vi "Set Matrix - file.vi"(5 "double array":dbl[][](array[numeric]), 6 "cmplx double array":cdb[][](array[numeric]), 7 "string array":string[](array[string]), 8 "error in (no error)":errorcluster, 10 "variable name":string, 11 "GOLPI ref. in":T1={"pipe handle"={"lv_proc.dll file path"=path "", "process instance handle"=[]}, "fast read timeout [ms]"=500, "fast read settle time [ms]"=10, "fast read to multiple [ms]"=1, "max elements per input line"=100}) -> (0 "error out":errorcluster, 3 "GOLPI ref. out":T1={"pipe handle"={"lv_proc.dll file path"=path "", "process instance handle"=[]}, "fast read timeout [ms]"=500, "fast read settle time [ms]"=10, "fast read to multiple [ms]"=1, "max elements per input line"=100})   [LabVIEW 2013, in "GOLPI library.lvlib"]
uses:
  GOLPI library.lvlib
  Type Definitions/GOLPI reference Type Def.ctl
  LV Process.lvlibp/Pipe Handle.ctl
  Type Definitions/Custom Error Codes Enum Type Def.vi
  LV Process.lvlibp
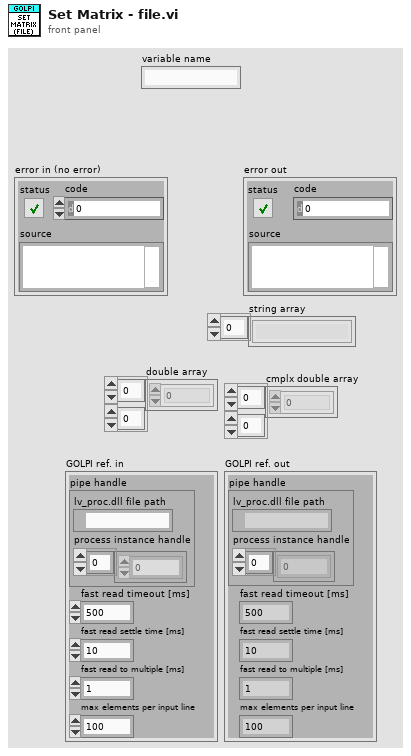
[diagram p1: front panel]
types:
  T1 = typedef "GOLPI library.lvlib/GOLPI reference Type Def.ctl" = cluster{"pipe handle":T2, "fast read timeout [ms]":u32, "fast read settle time [ms]":u32, "fast read to multiple [ms]":u32, "max elements per input line":u32}
  T2 = typedef "LV Process.lvlibp/Pipe Handle.ctl" = cluster{"lv_proc.dll file path":path, "process instance handle":u32[]}
  T3 = typedef "GOLPI library.lvlib/Custom Error Codes Enum Type Def.vi" = enum16{"no error", "00 working directory PAR1 missing", "01 octave binary PAR1 missing", "02 octave report error PAR1", "03 empty output last cmd PAR1", "04 missing temporary file PAR1", "05 pwd PAR 1 not exist", "10 var PAR1 not string", "11 var PAR1 not num, scal, ~compl", "12 var PAR1 not num, scal, compl", "13 var PAR1 not num, vect, ~compl", "14 var PAR1 not num, vect, compl", "15 var PAR1 not num, mat, ~compl", "16 var PAR1 not num, mat, ~compl", "99 not finished"}
  T4 = enum16{"open", "replace", "create", "open or create", "replace or create", "replace or create with confirmation"}
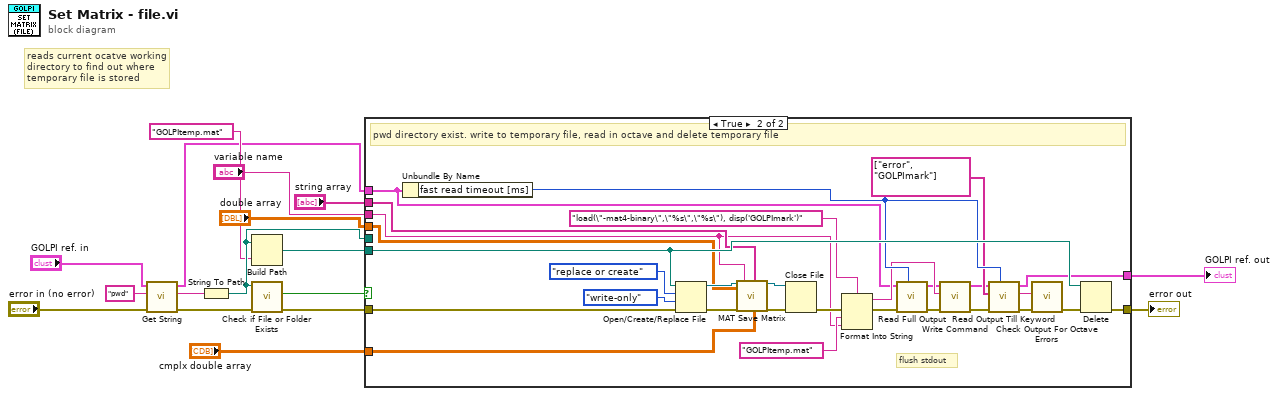
[diagram p0: block diagram]
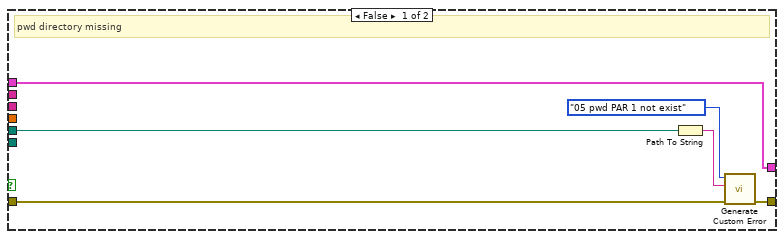
[diagram p2: hidden frame]
diagram:
  # "reads current ocatve working\ndirectory to find out where\ntemporary file is stored"
  n1 = call "Get String.vi"("error in"="error in (no error)", "variable name"="pwd", "GOLPI ref. in"="GOLPI ref. in") -> ("error out"=w7:errorcluster, "value"=w5:string, "GOLPI ref. out"=w1:T1)  [unwired: 6 in]
  n2 = String To Path(string=w5) -> (path=w3:path)
  n3 = Build Path(base path=w3, name or relative path="GOLPItemp.mat") -> (appended path=w4:path)
  n4 = call <vilib>:"Check if File or Folder Exists.vi"("error in (no error)"=w7, "path"=w3) -> ("error out"=w9:errorcluster, "file or folder exists?"=w8:bool)  [unwired: 7 in, 1 out]
  n5 = case shown="True" w8 {
    tunnel: [w22 w50] -> w17
    tunnel: w9 -> [w23 w49]
    tunnel: w4 -> [_ w48]
    tunnel: w3 -> [w19 _]
    tunnel: "variable name" -> [_ w25]
    tunnel: "string array" -> [_ w43]
    tunnel: "double array" -> [_ w42]
    tunnel: "cmplx double array" -> [_ w41]
    tunnel: w1 -> [w18 w26]
    tunnel: [w18 w24] -> w10
    frame False {
      # "pwd directory missing"
      n6 = Path To String(path=w19) -> (string=w20:string)
      n7 = call "Generate Custom Error.vi"("error in"=w23, "PAR1"=w20, "GOLPI error"=Custom_Error_Codes_Enum_Type_Def.vi."05 pwd PAR 1 not exist" ("Enum")) -> ("error out"=w22:errorcluster)  [unwired: 8 in]
    }
    frame True {
      # "flush stdout"
      # "pwd directory exist. write to temporary file, read in octave and delete temporary file"
      n8 = Unbundle By Name(w26) -> ("fast read timeout [ms]"=w40:u32)
      n9 = Open/Create/Replace File(file path (use dialog)=w48, error in=w49, operation (0:open)=T4."replace or create", access (0:read/write)=enum16{"read/write", "read-only", "write-only"}."write-only") -> (refnum out=w47:refnum<file>, error out=w46:errorcluster)  [unwired: 2 in, 1 out]
      n10 = call "MAT Save Matrix.vi"("Ref Num"=w47, "DBL"=w42, "error in (no error)"=w46, "Matrix Name"=w25, "STR"=w43, "CDB"=w41) -> ("Dup Ref Num"=w44:refnum<file>, "error out"=w45:errorcluster)  [unwired: 12 in]
      n11 = Close File(refnum=w44, error in=w45) -> (error out=w28:errorcluster)  [unwired: 1 out]
      n12 = Format Into String(format string="load(\"-mat4-binary\",\"%s\",\"%s\"), disp('GOLPImark')", error in=w28, "GOLPItemp.mat" ("name or relative path"), w25) -> (resulting string=w37:string, error out=w31:errorcluster)  [unwired: 1 in]
      n13 = call "Read Full Output.vi"("timeout [ms]"=w40, "error in"=w31, "GOLPI ref. in"=w26) -> ("error out"=w30:errorcluster, "GOLPI ref. out"=w29:T1)  [unwired: 5 in, 2 out]
      n14 = call "Write Command.vi"("error in"=w30, "command"=w37, "GOLPI ref. in"=w29) -> ("error out"=w32:errorcluster, "GOLPI ref. out"=w35:T1)  [unwired: 7 in]
      n15 = call "Read Output Till Keyword.vi"("timeout [ms]"=w40, "error in"=w32, "keywords"=string[] ["error", "GOLPImark"], "GOLPI ref. in"=w35) -> ("error out"=w33:errorcluster, "read buffer"=w34:string, "GOLPI ref. out"=w24:T1)  [unwired: 4 in, 1 out]
      n16 = call "Check Output For Octave Errors.vi"("error in"=w33, "read buffer"=w34) -> ("error out"=w27:errorcluster)  [unwired: 9 in]
      n17 = Delete(path (use dialog)=w48, error in=w27) -> (error out=w50:errorcluster)  [unwired: 3 in, 2 out]
    }
  }
  "error out" <- w17
  "GOLPI ref. out" <- w10
